vi "Get Telnet Reference.vi"(8 "error in (no error)":errorcluster, 11 "niDTS Comm Telnet in":refnum<class "niDTS Comm Telnet.lvclass">) -> (0 "error out":errorcluster, 2 "telnet connection refnum":T1, 3 "niDTS Comm Telnet out":refnum<class "niDTS Comm Telnet.lvclass">)   [LabVIEW 2015, in "niDTS CommLib.lvlib" / "niDTS Comm Telnet.lvclass"]
uses:
  niDTS Comm Telnet.lvclass
  Utility/telnet/telnet.llb/Telnet Session.ctl
  niDTS Comm Telnet.lvclass/niDTS Comm Telnet.ctl
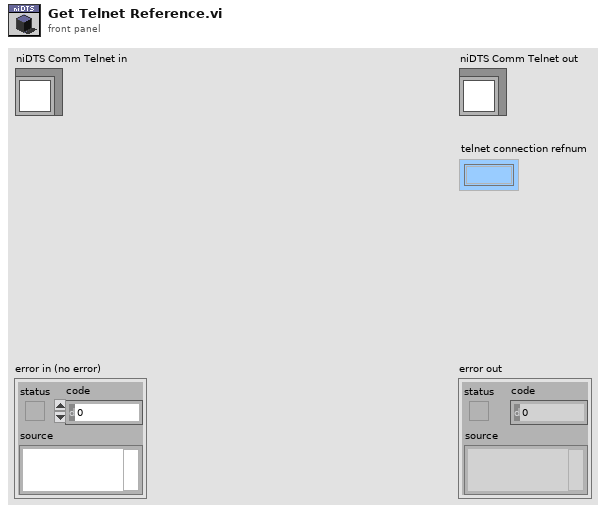
[diagram p1: front panel]
types:
  T1 = typedef "Telnet Session.ctl" = refnum<k1>
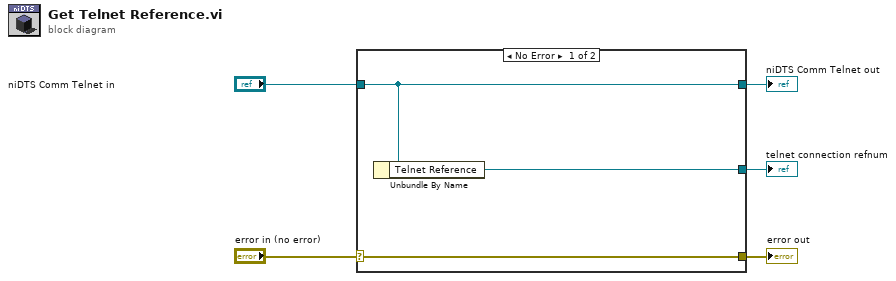
[diagram p0: block diagram]
diagram:
  n1 = case shown="No Error" "error in (no error)" {
    selector: "error in (no error)" -> [w8 w9]
    tunnel: [w8 w9] -> w4
    tunnel: [w7 w10] -> w2
    tunnel: "niDTS Comm Telnet in" -> [w7 w10]
    tunnel: [w6 _] -> w1
    frame No Error {
      n2 = Unbundle By Name(w7) -> ("Telnet Reference"=w6:T1)
    }
    frame Error {
    }
  }
  "error out" <- w4
  "niDTS Comm Telnet out" <- w2
  "telnet connection refnum" <- w1
